vi "AWG Setup for Butterfly.vi"(6 "AmpGain":dbl, 8 "error in (no error)":errorcluster, 9 "DOWNVoltages":dbl[](array[numeric]), 10 "UPVoltages":dbl[](array[numeric]), 11 "Semiconductor Module Context in":T1) -> (0 "error out":errorcluster, 1 "DOWNPublishNames":string[](array[string]), 2 "UPPublishNames":string[](array[string]), 3 "Semiconductor Module Context out":T1, 4 "Down_Butterfly_V_Sweep":dbl[](array[numeric]), 5 "Up_Butterfly_V_Sweep":dbl[](array[numeric]))   [LabVIEW 2013]
uses:
  <vilib>/NI_TestStand_SemiconductorModule/NI_TestStand_Semiconductor_Module.lvlibp/PinMap/General/SemiconductorModuleContext.ctl
  <vilib>/NI_TestStand_SemiconductorModule/NI_TestStand_Semiconductor_Module.lvlibp
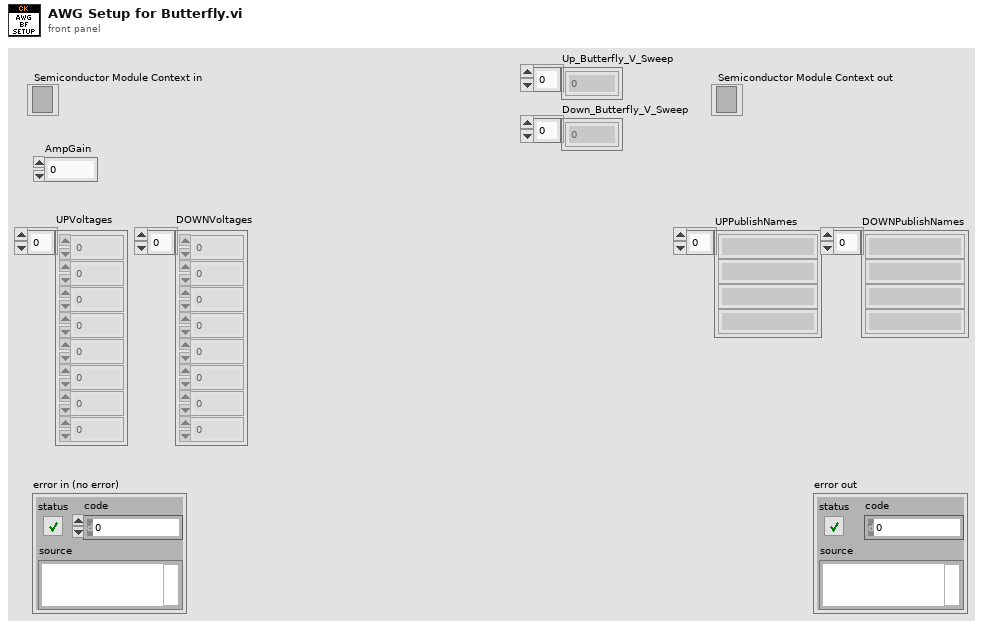
[diagram p1: front panel]
types:
  T1 = typedef "NI_TestStand_Semiconductor_Module.lvlibp/SemiconductorModuleContext.ctl" = refnum<k7>
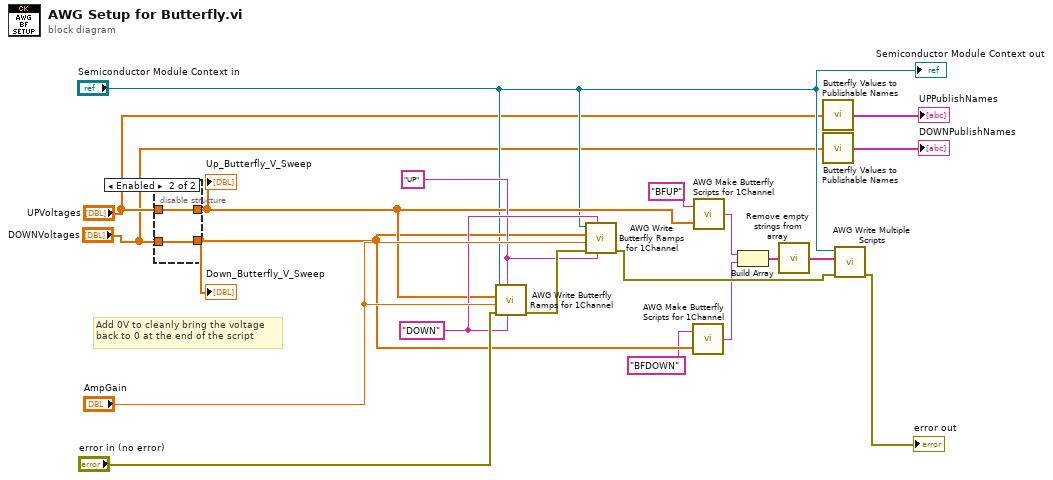
[diagram p0: block diagram]
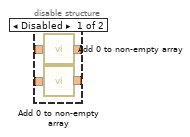
[diagram p2: hidden frame]
diagram:
  w17 = "DOWN" ("Secondary Pin Name")
  w16 = "UP" ("Main Pin Name")
  # "Add 0V to cleanly bring the voltage\nback to 0 at the end of the script"
  n1 = disable-structure shown="Enabled" {
    disable-tunnel: [w24 w26] -> w15
    disable-tunnel: [w23 w25] -> w14
    disable-tunnel: "UPVoltages" -> [w22 w26]
    disable-tunnel: "DOWNVoltages" -> [w21 w25]
    frame Disabled {
      n2 = call "Add 0 to non-empty array.vi"("Voltages in"=w22) -> ("Voltages out"=w24:dbl[])
      n3 = call "Add 0 to non-empty array.vi"("Voltages in"=w21) -> ("Voltages out"=w23:dbl[])
    }
    frame Enabled {
    }
  }
  "Up_Butterfly_V_Sweep" <- w15
  "Down_Butterfly_V_Sweep" <- w14
  n4 = call "AWG Write Butterfly Ramps for 1Channel.vi"("Secondary Pin Name"=w17, "Main Pin Name"=w16, "error in (no error)"="error in (no error)", "AmpGain"="AmpGain", "Voltages"=w15, "Automation Refnum in"="Semiconductor Module Context in") -> ("error out"=w19:errorcluster)  [unwired: 5 in]
  n5 = call "AWG Write Butterfly Ramps for 1Channel.vi"("Secondary Pin Name"=w16, "Main Pin Name"=w17, "error in (no error)"=w19, "AmpGain"="AmpGain", "Voltages"=w14, "Automation Refnum in"="Semiconductor Module Context in") -> ("error out"=w11:errorcluster)  [unwired: 5 in]
  n6 = call "AWG Make Butterfly Scripts for 1Channel.vi"("Voltages"=w14, "Prefix"="BFDOWN") -> ("String"=w9:string)
  n7 = call "AWG Make Butterfly Scripts for 1Channel.vi"("Voltages"=w15, "Prefix"="BFUP") -> ("String"=w8:string)
  n8 = Build Array(w8, w9) -> (w2:string[])
  n9 = call "Remove empty strings from array.vi"("Array in"=w2) -> ("Array out"=w1:string[])
  n10 = call "Butterfly Values to Publishable Names.vi"("Butterfly Numbers"="UPVoltages") -> ("Publishable Names"=→"UPPublishNames":string[])
  n11 = call "Butterfly Values to Publishable Names.vi"("Butterfly Numbers"="DOWNVoltages") -> ("Publishable Names"=→"DOWNPublishNames":string[])
  n12 = call "AWG Write Multiple Scripts.vi"("error in"=w11, "Scripts"=w1, "Semiconductor Module Context"="Semiconductor Module Context in") -> ("error out"=→"error out":errorcluster)  [unwired: 8 in]
  "Semiconductor Module Context out" <- "Semiconductor Module Context in"
